vi "Send List of Functions Message.vi"(8 "error in (no error)":errorcluster, 10 "List of Function Names":string[](array[string]), 11 "Message Enqueuer in":refnum<class "Message Enqueuer.lvclass">) -> (0 "error out":errorcluster, 3 "Message Enqueuer out":refnum<class "Message Enqueuer.lvclass">)   [LabVIEW 2016, in "Controller UI.lvlib" / "List of Functions Message.lvclass"]
uses:
  <userlib>/Common Components/Controller UI/Messages/List of Functions Message/List of Functions Message.lvclass
  <vilib>/ActorFramework/Message Enqueuer/Message Enqueuer.lvclass
  C:/Program Files (x86)/National Instruments/LabVIEW 2016/vi.lib/ActorFramework/Message/Message.lvclass
  <vilib>/ActorFramework/Message Enqueuer/Message Enqueuer.lvclass/Message Enqueuer.ctl
  <vilib>/ActorFramework/Message Priority Queue/Priority Enqueue.vi
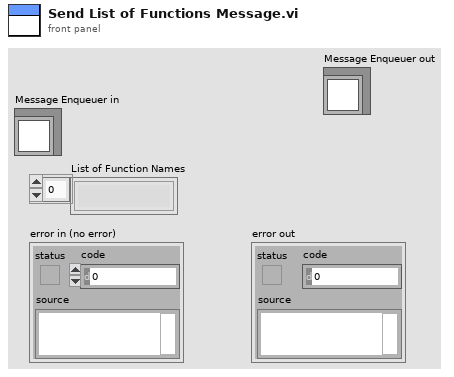
[diagram p1: front panel]
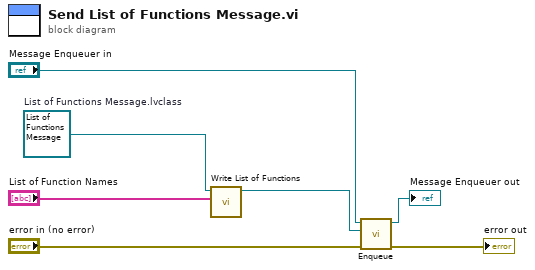
[diagram p0: block diagram]
diagram:
  w7 = refnum<class "List of Functions Message.lvclass"> refnum  # List of Functions Message.lvclass
  n1 = call <userlib>:"Write List of Functions.vi"("List of Functions"="List of Function Names", "List of Functions Message in"=w7) -> ("List of Functions Message out"=w3:refnum<class "List of Functions Message.lvclass">)  [unwired: 8 in, 1 out]
  n2 = call <vilib>:"Enqueue.vi"("error in (no error)"="error in (no error)", "Message"=w3, "Message Enqueuer in"="Message Enqueuer in") -> ("error out"=→"error out":errorcluster, "Message Enqueuer out"=→"Message Enqueuer out":refnum<class "Message Enqueuer.lvclass">)  [unwired: 7 in]
